vi "Init.vi"(8 "error in (no error)":errorcluster, 10 "WindowTitle":string, 11 "WindowFrame in":refnum<class "WindowFrame.lvclass">) -> (0 "error out":errorcluster, 2 "WindowFrame":refnum<event-registration>, 3 "WindowFrame out":refnum<class "WindowFrame.lvclass">)   [LabVIEW 2021, in "WindowFrame.lvlib" / "WindowFrame.lvclass"]
uses:
  WindowFrame.lvclass
  WindowFrame.lvclass/WindowFrame.ctl
  Action.ctl
  ActionData.ctl
  75890353-0d9d-4771-b0d2-9ab8773a2eba.vi
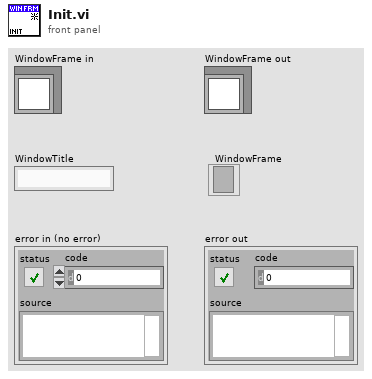
[diagram p1: front panel]
types:
  T1 = typedef "WindowFrame.lvlib/WindowFrame.lvclass/ActionData.ctl" = cluster{"Action":T2, "Variant":variant}
  T2 = typedef "WindowFrame.lvlib/WindowFrame.lvclass/Action.ctl" = enum16{"Set Allow Runtime PopUp", "Set Behavior", "Set Closable", "Set Custom Title", "Set Highlight Return Button", "Set Is Frontmost", "Set Minimizable", "Set Minimum Size", "Set Monitor", "Set Resizable", "Set Panel Bounds", "Set Run VI Transparently", "Set Show Menu Bar", "Set State", "Set Title", "Set Title Bar Colors", "Set Title Bar Visible", "Set Transparancy", "Set Window Bounds", "Get Allow Runtime PopUp", "Get Behavior", "Get Closable", "Get Custom Title", "Get Highlight Return Button", "Get Is Frontmost", "Get Minimizable", "Get Minimum Size", "Get Monitor", "Get Panel Bounds", "Get Resizable", "Get Run VI Transparently", "Get Show Menu Bar", "Get State", "Get Title", "Get Title Bar Colors", "Get Title Bar Visible", "Get Transparancy", "Get Window Bounds", "--", "Center", "Close", "Open", "Run-Time Position:Centered", "Run-Time Position:Custom", "Run-Time Position:Get Position", "Run-Time Position:Maximized", "Run-Time Position:Minimized", "Run-Time Position:Unchanged", "---", "Insert VI", "Remove VI", "Insert VI Index", "Remove VI Index", "Exit"}
  T3 = enum32{"Invalid", "Standard", "Closed", "Hidden", "Minimized", "Maximized"}
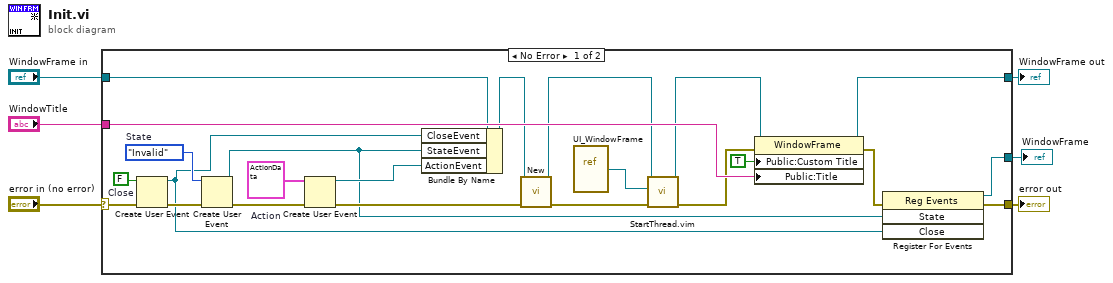
[diagram p0: block diagram]
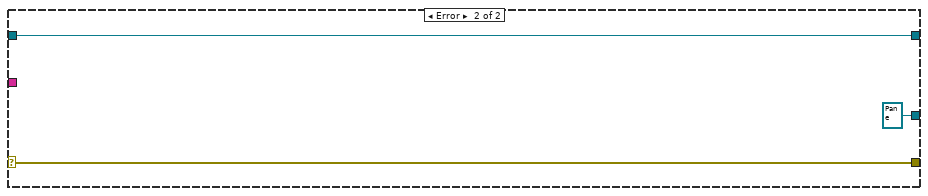
[diagram p2: hidden frame]
diagram:
  n1 = case shown="No Error" "error in (no error)" {
    selector: "error in (no error)" -> [w10 w32]
    tunnel: [w18 w31] -> w6
    tunnel: "WindowTitle" -> [w29 _]
    tunnel: [w23 w32] -> w4
    tunnel: [w22 refnum<event-registration> refnum ("Event Registration Refnum")] -> w1
    tunnel: "WindowFrame in" -> [w16 w31]
    frame No Error {
      w8 = FALSE  # Close
      w26 = T1 {"Action"=enum."Set Allow Runtime PopUp", "Variant"=variant}  # Action
      w20 = T3."Invalid"  # State
      n2 = Create User Event(user event datatype=w8, error in=w10) -> (user event=w7:refnum<user-event>, error out=w9:errorcluster)
      n3 = Create User Event(user event datatype=w20, error in=w9) -> (user event=w21:refnum<user-event>, error out=w24:errorcluster)
      n4 = Create User Event(user event datatype=w26, error in=w24) -> (user event=w27:refnum<user-event>, error out=w25:errorcluster)
      n5 = Bundle By Name(cluster=w16, "CloseEvent"=w7, "StateEvent"=w21, "ActionEvent"=w27) -> (w17:refnum<class "WindowFrame.lvclass">)
      n6 = call-dynamic "New.vi"("error in (no error)"=w25, "ByRefClass in"=w17) -> ("error out"=w15:errorcluster, "ByRefClass out"=w13:refnum<class "WindowFrame.lvclass">)  [unwired: 8 in]
      n7 = vi-ref "UI_WindowFrame.vi"() -> (w14:refnum<vi>)
      n8 = call "StartThread.vim"("error in (no error)"=w15, "VI Refnum in"=w14, "ByRefClass in"=w13) -> ("error out"=w11:errorcluster, "ByRefClass out"=w12:refnum<class "WindowFrame.lvclass">)  [unwired: 6 in, 1 out]
      n9 = property class="WindowFrame"(reference=w12, error in=w11, "Public:Custom Title"=TRUE ("Custom Title"), "Public:Title"=w29) -> (reference out=w18:refnum<class "WindowFrame.lvclass">, error out=w28:errorcluster)
      n10 = register-events(error in=w28, w21, w7) -> (reference out=w22:refnum<event-registration>, error out=w23:errorcluster)  [unwired: 1 in]
    }
    frame Error {
    }
  }
  "WindowFrame out" <- w6
  "error out" <- w4
  "WindowFrame" <- w1
